vi "THD_Mess_Status.vi"() -> ()   [LabVIEW 2018]
panel:
  out "Boolean":bool
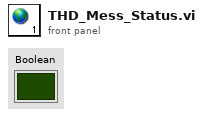
[diagram p1: front panel]
diagram:
